vi "SignalGenAdq_Activity 2.vi"() -> ()   [LabVIEW 2015]
panel:
  out "Waveform Chart 2":dynamicdata(graph)
  out "Waveform Chart":dbl(graph)
  in  "stop":bool
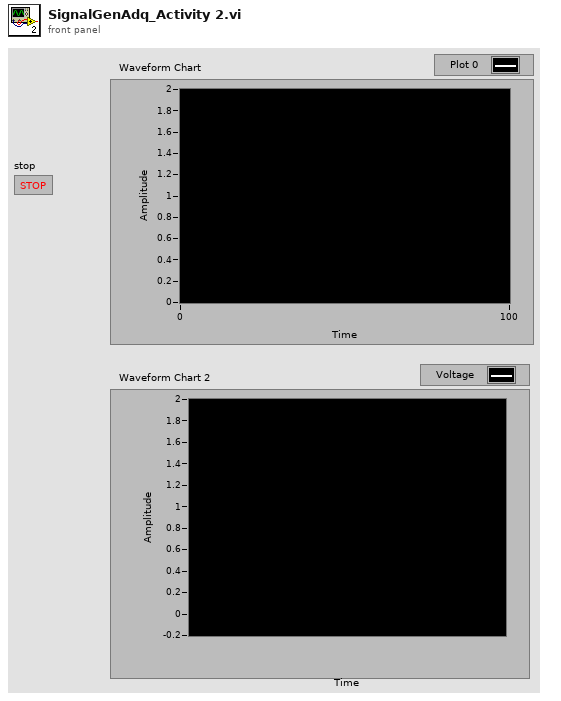
[diagram p1: front panel]
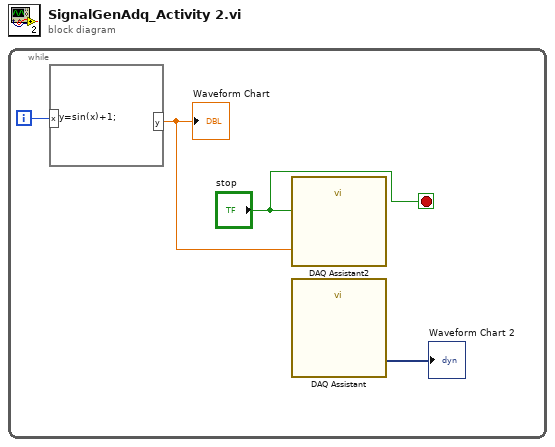
[diagram p0: block diagram]
diagram:
  n1 = while {
    i -> [w4]
    stop <- "stop" stop-if-true
    n2 = formula code="y=sin(x)+1;"("x"=w4) -> ("y"=w2:dbl)
    "Waveform Chart" <- w2
    n3 = call "DAQ Assistant2"("data"=w2, "stop (T)"="stop") -> ()  [unwired: 16 in, 2 out]
    n4 = call "DAQ Assistant"() -> ("data"=→"Waveform Chart 2":dynamicdata)  [unwired: 16 in, 3 out]
  }
